vi "Grove I2C LCD Class.vi"() -> ()   [LabVIEW 2020]
uses:
  CTI-Peripheral/Grove I2C LCD/Grove I2C LCD.lvclass
panel:
  in  "Grove I2C LCD":refnum<class "Grove I2C LCD.lvclass">
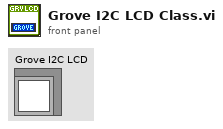
[diagram p1: front panel]
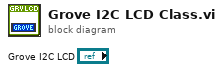
[diagram p0: block diagram]
diagram:
